vi "Exponential Fit Coefficients PtByPt.vi"(0 "y":dbl format="%0.2f", 1 "x":dbl format="%0.2f", 3 "sample length":i32=100, 4 "initialize":bool) -> (5 "History of x":dbl[](array[numeric]), 6 "History of y":dbl[](array[numeric]), 7 "amplitude":dbl format="%0.2f", 8 "damping":dbl format="%0.2f", 10 "error":i32)   [LabVIEW 2017, in "NI_PtbyPt.lvlib"]
doc: "Finds the exponential coefficients <B>amplitude</B> and <B>damping</B>, using the least-squares solution, which describe the exponential curve that best represents the set of input data points specified by <B>sample length</B>."
uses:
  <vilib>/ptbypt/NI_PtbyPt.lvlib
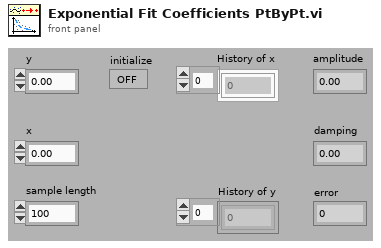
[diagram p1: front panel]
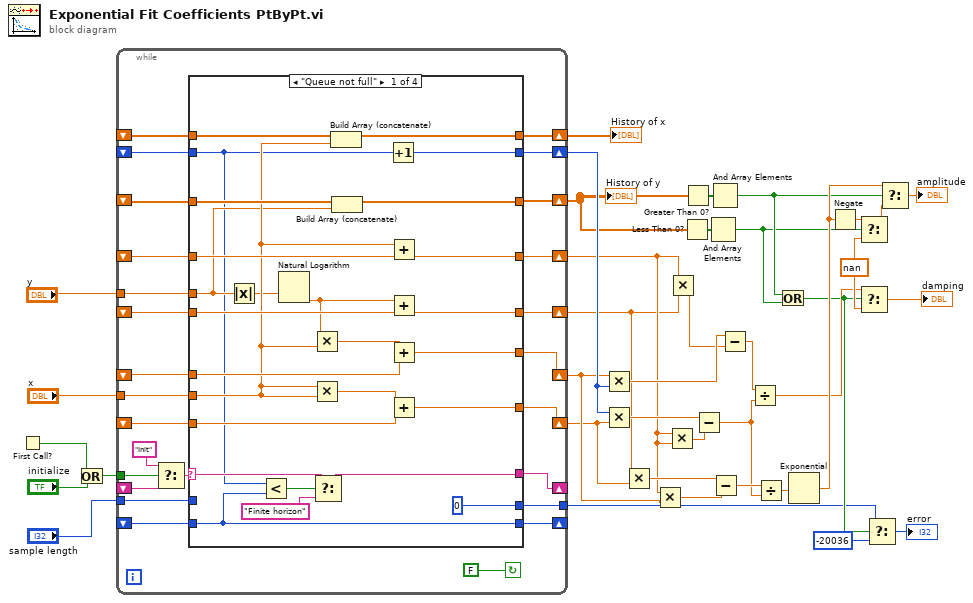
[diagram p0: block diagram]
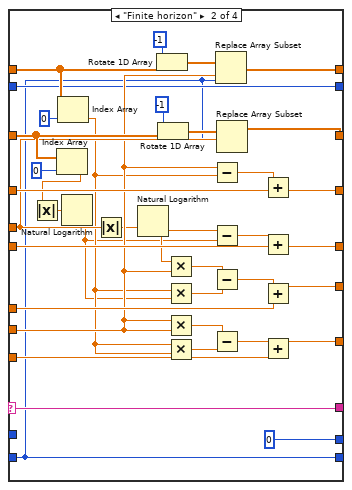
[diagram p2: hidden frame]
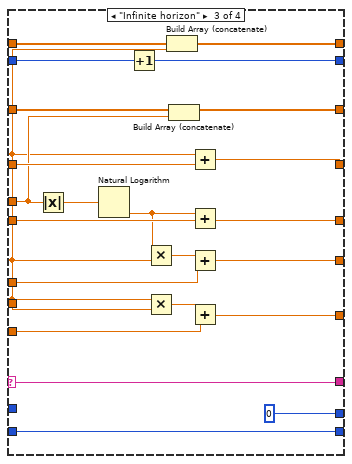
[diagram p3: hidden frame]
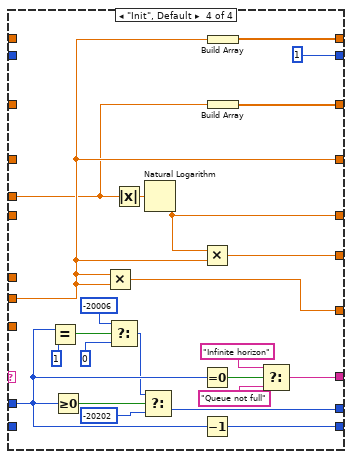
[diagram p4: hidden frame]
diagram:
  w11 = nan ("f")
  n1 = First Call?() -> (First Call?: T/F=w19:bool)
  n2 = Or(x=w19, y="initialize") -> (x .or. y?=w17:bool)
  n3 = while {
    tunnel: [w39] -> w1
    shift-left: _ -> [w44]
    shift-right: [w48] -> _
    shift-left: _ -> [w49]
    shift-right: [w47] -> _
    tunnel: w17 -> [w50]
    shift-left: _ -> [w54]
    shift-right: [w53] -> w25
    shift-left: _ -> [w55]
    shift-right: [w56] -> w26
    tunnel: "y" -> [w40]
    shift-left: _ -> [w58]
    shift-right: [w57] -> w27
    shift-left: _ -> [w59]
    shift-right: [w42] -> w28
    shift-left: _ -> [w60]
    shift-right: [w41] -> w14
    shift-left: _ -> [w61]
    shift-right: [w45] -> w29
    tunnel: "x" -> [w62]
    tunnel: "sample length" -> [w64]
    shift-left: _ -> [w63]
    shift-right: [w46] -> w20
    stop <- FALSE continue-if-true
    n4 = Select(t="Init", s=w50, f=w49) -> (s? t:f=w52:string)
    n5 = case shown="\"Queue not full\"" w52 {
      selector: w52 -> [w77 w98 w145 _]
      tunnel: w62 -> [w74 w105 w135 w163]
      tunnel: w64 -> [_ _ _ w171]
      tunnel: [w81 w127 w150 w164] -> w46
      tunnel: w63 -> [w82 w122 w151 _]
      tunnel: w61 -> [w68 w97 w149 _]
      tunnel: w60 -> [w80 w120 w147 _]
      tunnel: [w79 w123 w146 w167] -> w41
      tunnel: [w89 w116 w142 w163] -> w42
      tunnel: w59 -> [w90 w117 w143 _]
      tunnel: w40 -> [w73 w112 w137 w161]
      tunnel: w58 -> [w88 w114 w141 _]
      tunnel: [w87 w113 w140 w160] -> w57
      tunnel: [w86 w106 w138 w174] -> w56
      tunnel: w55 -> [w85 w107 w139 _]
      tunnel: w54 -> [w84 w100 w133 _]
      tunnel: [w83 w99 w132 w162] -> w53
      tunnel: [w70 w96 w144 w166] -> w48
      tunnel: [w76 w98 w145 w168] -> w47
      tunnel: [w69 w97 w148 1] -> w45
      tunnel: w44 -> [w70 w96 w144 _]
      tunnel: [0 ("f") 0 ("f") 0 ("f") w152] -> w39
      frame "Queue not full" {
        n6 = Absolute Value(x=w73) -> (abs(x)=w66:dbl)
        n7 = Less?(x=w68, y=w70) -> (x < y?=w78:bool)
        n8 = Natural Logarithm(1:w66) -> (0:w67:dbl)
        n9 = Multiply(x=w67, y=w74) -> (x*y=w72:dbl)
        n10 = Multiply(x=w74, y=w74) -> (x*y=w71:dbl)
        n11 = Select(t=w77, s=w78, f="Finite horizon") -> (s? t:f=w76:string)
        n12 = Build Array (concatenate)(w82, w74) -> (w81:dbl[])
        n13 = Build Array (concatenate)(w80, w73) -> (w79:dbl[])
        n14 = Increment(x=w68) -> (x+1=w69:i32)
        n15 = Add(x=w74, y=w90) -> (x+y=w89:dbl)
        n16 = Add(x=w67, y=w88) -> (x+y=w87:dbl)
        n17 = Add(x=w72, y=w85) -> (x+y=w86:dbl)
        n18 = Add(x=w71, y=w84) -> (x+y=w83:dbl)
      }
      frame "Finite horizon" {
        n19 = Index Array(array=w120, index=0 ("Index")) -> (element=w111:dbl)
        n20 = Absolute Value(x=w111) -> (abs(x)=w93:dbl)
        n21 = Index Array(array=w122, index=0 ("Index")) -> (element=w104:dbl)
        n22 = Natural Logarithm(1:w93) -> (0:w94:dbl)
        n23 = Absolute Value(x=w112) -> (abs(x)=w92:dbl)
        n24 = Natural Logarithm(1:w92) -> (0:w95:dbl)
        n25 = Rotate 1D Array(1:w122, 2:i16 -1 ("n")) -> (0:w126:dbl[])
        n26 = Rotate 1D Array(1:w120, 2:i16 -1 ("n")) -> (0:w124:dbl[])
        n27 = Multiply(x=w95, y=w105) -> (x*y=w110:dbl)
        n28 = Multiply(x=w104, y=w94) -> (x*y=w109:dbl)
        n29 = Multiply(x=w105, y=w105) -> (x*y=w103:dbl)
        n30 = Multiply(x=w104, y=w104) -> (x*y=w102:dbl)
        n31 = Subtract(x=w105, y=w104) -> (x-y=w118:dbl)
        n32 = Subtract(x=w95, y=w94) -> (x-y=w115:dbl)
        n33 = Subtract(x=w110, y=w109) -> (x-y=w108:dbl)
        n34 = Subtract(x=w103, y=w102) -> (x-y=w101:dbl)
        n35 = Replace Array Subset(array=w126, new element=w105, index=w96) -> (w127:dbl[])
        n36 = Replace Array Subset(array=w124, new element=w112, index=w96) -> (w123:dbl[])
        n37 = Add(x=w118, y=w117) -> (x+y=w116:dbl)
        n38 = Add(x=w115, y=w114) -> (x+y=w113:dbl)
        n39 = Add(x=w108, y=w107) -> (x+y=w106:dbl)
        n40 = Add(x=w101, y=w100) -> (x+y=w99:dbl)
      }
      frame "Infinite horizon" {
        n41 = Absolute Value(x=w137) -> (abs(x)=w130:dbl)
        n42 = Natural Logarithm(1:w130) -> (0:w131:dbl)
        n43 = Increment(x=w149) -> (x+1=w148:i32)
        n44 = Multiply(x=w131, y=w135) -> (x*y=w136:dbl)
        n45 = Multiply(x=w135, y=w135) -> (x*y=w134:dbl)
        n46 = Build Array (concatenate)(w151, w135) -> (w150:dbl[])
        n47 = Build Array (concatenate)(w147, w137) -> (w146:dbl[])
        n48 = Add(x=w135, y=w143) -> (x+y=w142:dbl)
        n49 = Add(x=w131, y=w141) -> (x+y=w140:dbl)
        n50 = Add(x=w136, y=w139) -> (x+y=w138:dbl)
        n51 = Add(x=w134, y=w133) -> (x+y=w132:dbl)
      }
      frame "Init", Default {
        n52 = Equal?(x=w171, y=1) -> (x = y?=w157:bool)
        n53 = Greater Or Equal To 0?(x=w171) -> (x >= 0?=w156:bool)
        n54 = Multiply(x=w163, y=w163) -> (x*y=w162:dbl)
        n55 = Select(t=-20006 ("f"), s=w157, f=0) -> (s? t:f=w154:i32)
        n56 = Absolute Value(x=w161) -> (abs(x)=w153:dbl)
        n57 = Select(t=w154, s=w156, f=-20202) -> (s? t:f=w152:i32)
        n58 = Natural Logarithm(1:w153) -> (0:w160:dbl)
        n59 = Multiply(x=w160, y=w163) -> (x*y=w174:dbl)
        n60 = Equal To 0?(x=w171) -> (x = 0?=w173:bool)
        n61 = Decrement(x=w171) -> (x-1=w166:i32)
        n62 = Build Array(w163) -> (w164:dbl[])
        n63 = Build Array(w161) -> (w167:dbl[])
        n64 = Select(t="Infinite horizon", s=w173, f="Queue not full") -> (s? t:f=w168:string)
      }
    }
  }
  "History of x" <- w20
  "History of y" <- w14
  n65 = Multiply(x=w26, y=w29) -> (x*y=w38:dbl)
  n66 = Multiply(x=w29, y=w25) -> (x*y=w36:dbl)
  n67 = Multiply(x=w27, y=w25) -> (x*y=w33:dbl)
  n68 = Multiply(x=w28, y=w26) -> (x*y=w32:dbl)
  n69 = Multiply(x=w28, y=w28) -> (x*y=w35:dbl)
  n70 = Multiply(x=w28, y=w27) -> (x*y=w37:dbl)
  n71 = Less Than 0?(x=w14) -> (x < 0?=w16:bool[])
  n72 = Greater Than 0?(x=w14) -> (x > 0?=w15:bool[])
  n73 = Subtract(x=w36, y=w35) -> (x-y=w30:dbl)
  n74 = And Array Elements(Boolean array=w16) -> (logical AND=w7:bool)
  n75 = And Array Elements(Boolean array=w15) -> (logical AND=w8:bool)
  n76 = Subtract(x=w33, y=w32) -> (x-y=w31:dbl)
  n77 = Subtract(x=w38, y=w37) -> (x-y=w34:dbl)
  n78 = Divide(x=w34, y=w30) -> (x/y=w6:dbl)
  n79 = Divide(x=w31, y=w30) -> (x/y=w21:dbl)
  n80 = Or(x=w8, y=w7) -> (x .or. y?=w4:bool)
  n81 = Exponential(1:w21) -> (0:w10:dbl)
  n82 = Negate(x=w10) -> (-x=w13:dbl)
  n83 = Select(t=w13, s=w7, f=w11) -> (s? t:f=w12:dbl)
  n84 = Select(t=w6, s=w4, f=w11) -> (s? t:f=→"damping":dbl)
  n85 = Select(t=w1, s=w4, f=-20036) -> (s? t:f=→"error":i32)
  n86 = Select(t=w10, s=w8, f=w12) -> (s? t:f=→"amplitude":dbl)
